vi "Integral.vi"(11 "Aceleração atual":dbl) -> (0 "Old aceleração":dbl, 3 "Posição":dbl format="%#_6f")   [LabVIEW 2016]
panel:
  out "double precision float":dbl
  out "Aceleração atual 2":dbl
  out "último tempo":dbl
  out "Old Velocidade":dbl format="%#_6f"
  out "Old Time":dbl
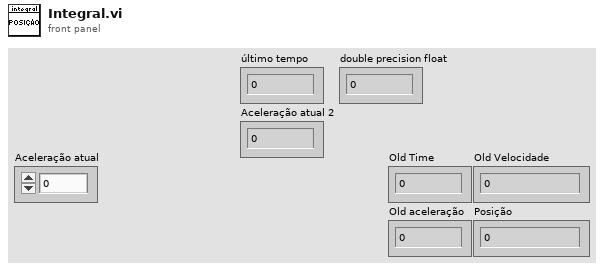
[diagram p1: front panel]
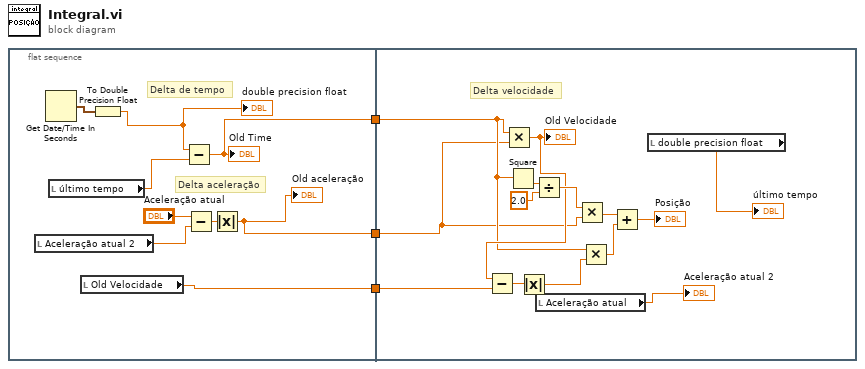
[diagram p0: block diagram]
diagram:
  n1 = flat-sequence {
    tunnel: [w11] -> w3
    tunnel: [w10] -> w2
    tunnel: [w9] -> w1
    tunnel: w3 -> [w21]
    tunnel: w2 -> [w16]
    tunnel: w1 -> [w17]
    frame #0 {
      # "Delta aceleração"
      # "Delta de tempo"
      n2 = local read "Aceleração atual 2"() -> (w4:dbl)
      n3 = Get Date/Time In Seconds() -> (seconds since 1Jan1904=w8:timestamp)
      n4 = local read "último tempo"() -> (w5:dbl)
      n5 = local read "Old Velocidade"() -> (w11:dbl)
      n6 = To Double Precision Float(number=w8) -> (double precision float=w7:dbl)
      "double precision float" <- w7
      n7 = Subtract(x=w7, y=w5) -> (x-y=w9:dbl)
      "Old Time" <- w9
      n8 = Subtract(x="Aceleração atual", y=w4) -> (x-y=w12:dbl)
      n9 = Absolute Value(x=w12) -> (abs(x)=w10:dbl)
      "Old aceleração" <- w10
    }
    frame #1 {
      # "Delta velocidade"
      n10 = Multiply(x=w17, y=w16) -> (x*y=w22:dbl)
      "Old Velocidade" <- w22
      n11 = Subtract(x=w22, y=w21) -> (x-y=w15:dbl)
      n12 = Square(x=w17) -> (x^2=w26:dbl)
      n13 = Absolute Value(x=w15) -> (abs(x)=w20:dbl)
      n14 = Divide(x=w26, y=2.0) -> (x/y=w24:dbl)
      n15 = local read "Aceleração atual"() -> (→"Aceleração atual 2":dbl)
      n16 = Multiply(x=w24, y=w16) -> (x*y=w23:dbl)
      n17 = Multiply(x=w17, y=w20) -> (x*y=w19:dbl)
      n18 = Add(x=w23, y=w19) -> (x+y=→"Posição":dbl)
      n19 = local read "double precision float"() -> (→"último tempo":dbl)
    }
  }
